vi "Set Select Platform Event.vi"(8 "error in (no error)":errorcluster, 10 "Select Platform Event":refnum<user-event>, 11 "PlatformArrayPanel in":refnum<class "PlatformArrayPanel.lvclass">) -> (0 "error out":errorcluster, 3 "PlatformArrayPanel out":refnum<class "PlatformArrayPanel.lvclass">)   [LabVIEW 2020, in "PicoG-App.lvlib" / "PlatformArrayPanel.lvclass"]
uses:
  PlatformArrayPanel.lvclass
  Builds/picoG/ppl/PicoG-Core.lvlibp/PicoG-Processor/PicoG-Core/Platform/Platform.lvclass
  PlatformArrayPanel.lvclass/PlatformArrayPanel.ctl
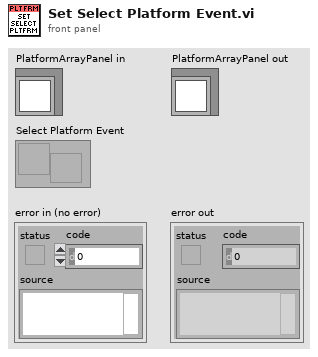
[diagram p1: front panel]
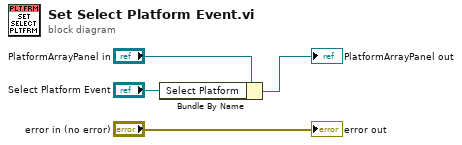
[diagram p0: block diagram]
diagram:
  n1 = Bundle By Name(cluster="PlatformArrayPanel in", "Select Platform"="Select Platform Event") -> (→"PlatformArrayPanel out":refnum<class "PlatformArrayPanel.lvclass">)
  "error out" <- "error in (no error)"
